vi "RT - Process Acquire Loop Error Flags.vi"(8 "error in (no error)":errorcluster, 11 "Error Flags":bool[](array[boolean])) -> (0 "error out":errorcluster)   [LabVIEW 2014]
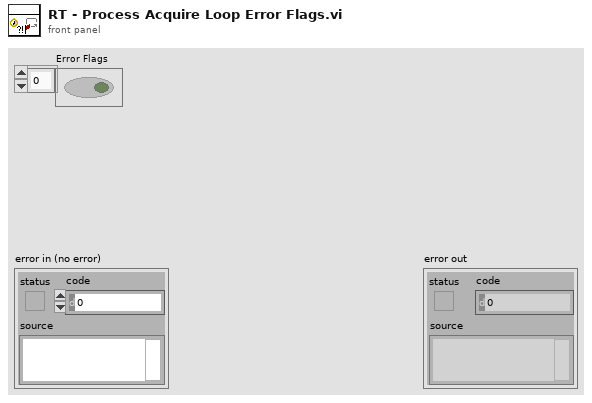
[diagram p1: front panel]
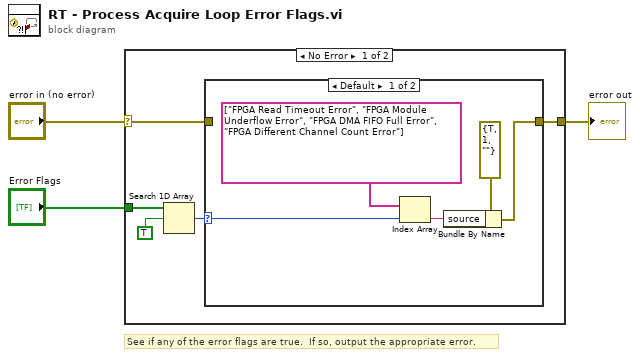
[diagram p0: block diagram]
diagram:
  # "See if any of the error flags are true.  If so, output the appropriate error."
  n1 = case shown="No Error" "error in (no error)" {
    selector: "error in (no error)" -> [w5 w15]
    tunnel: [w4 w15] -> w2
    tunnel: "Error Flags" -> [w8 _]
    frame No Error {
      n2 = Search 1D Array(1D array=w8, element=TRUE) -> (index of element=w6:i32)  [unwired: 1 in]
      n3 = case shown="Default" w6 {
        selector: w6 -> [w11 _]
        tunnel: w5 -> [_ w14]
        tunnel: [w12 w14] -> w4
        frame Default {
          n4 = Index Array(array=string[] ["FPGA Read Timeout Error", "FPGA Module Underflow Error", "FPGA DMA FIFO Full Error", "FPGA Different Channel Count Error"], index=w11) -> (element=w10:string)
          n5 = Bundle By Name(cluster=errorcluster {"status"=TRUE, "code"=1, "source"=""} ("error constant"), "source"=w10) -> (w12:errorcluster)
        }
        frame -1 {
        }
      }
    }
    frame Error {
    }
  }
  "error out" <- w2
